vi "_CSMOFGV(lvlibp).vi"(6 "Operation":T7=enum."Get By Name", 7 "Allowed Messages (Empty For All)":string[](array[string]), 8 "Error In":errorcluster caption="error in (no error)", 9 "Mode":T1, 10 "Reference":string, 11 "Name (\"\" to Use UUID) In":string) -> (0 "error out":errorcluster, 1 "Boolean":bool, 3 "Array":T2[](array[typedef]))   [LabVIEW 2017, in "Communicable State Machine.lvlib"]
uses:
  Communicable State Machine.lvlib
  _CSMOFGVOPER.ctl
  _CSMObj.ctl
  _CSMObj-Info.ctl
  Typedef/_CSM_MODE.ctl
  _CSMObj-Refs.ctl
  _CSMObj-Data.ctl
  Typedef/_CSM_MSG_TYPE.ctl
  Priority Queue/Priority Queue.ctl
  Typedef/_Cross CSM State Data.ctl
  Typedef/_Cross CSM State Response.ctl
  Typedef/_CSM_Response Source Message.ctl
  Priority Queue/def-Data(LowPRI-Q).ctl
  _CSMObj-ModeData.ctl
  Typedef/_CSM Status Change Event Data.ctl
  Typedef/_CSM_List Module Scope.ctl
  _CSMOFGV.vi
  _Shared/CSM Shared.lvlib
panel:
  out "data":path
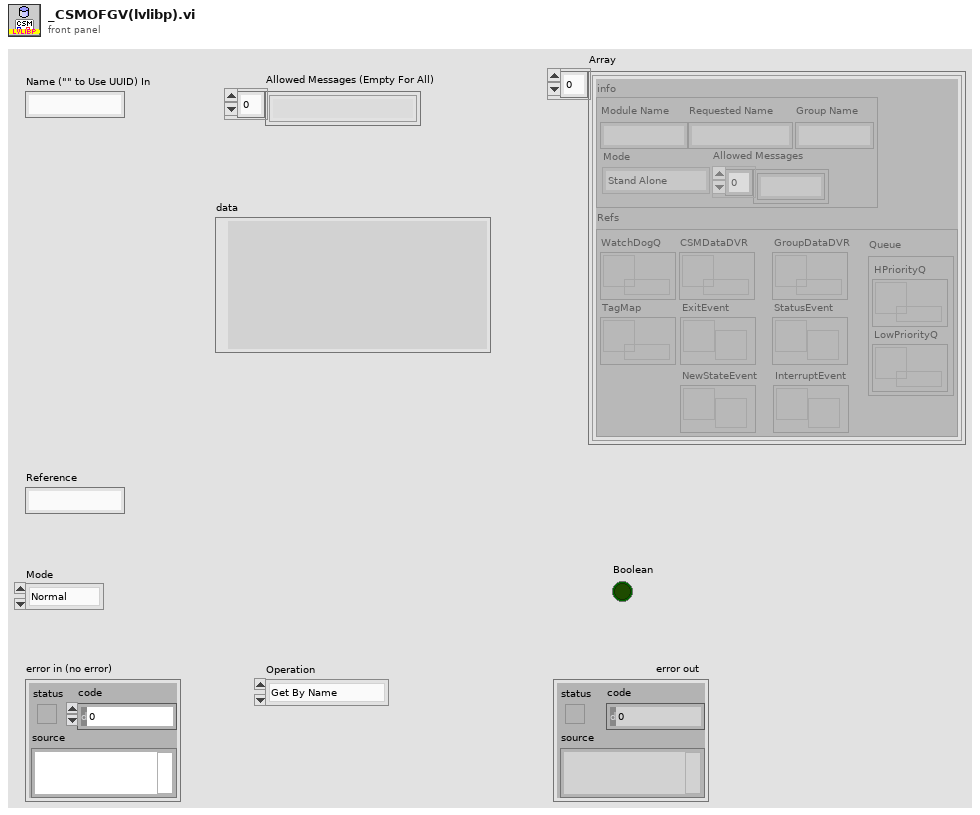
[diagram p1: front panel]
types:
  T1 = typedef "Communicable State Machine.lvlib/_CSM_List Module Scope.ctl" = enum16{"Normal", "System Only", "All"}
  T2 = typedef "Communicable State Machine.lvlib/_CSMObj.ctl" = cluster{"info":T3, "Refs":T5}
  T3 = typedef "Communicable State Machine.lvlib/_CSMObj-Info.ctl" = cluster{"Module Name":string, "Requested Name":string, "Group Name":string, "Mode":T4, "Allowed Messages":string[]}
  T4 = typedef "Communicable State Machine.lvlib/_CSM_MODE.ctl" = enum16{"Not Exist", "Stand Alone", "CSM", "Worker", "Worker Agent", "Chain Node", "Chain"}
  T5 = typedef "Communicable State Machine.lvlib/_CSMObj-Refs.ctl" = cluster{"WatchDogQ":refnum<queue>, "CSMDataDVR":refnum<data-value>, "Queue":T6, "GroupDataDVR":refnum<data-value>, "TagMap":refnum<data-value>, "ExitEvent":refnum<user-event>, "NewStateEvent":refnum<user-event>, "StatusEvent":refnum<user-event>, "InterruptEvent":refnum<user-event>}
  T6 = typedef "Communicable State Machine.lvlib/Priority Queue.ctl" = cluster{"HPriorityQ":refnum<queue>, "LowPriorityQ":refnum<queue>}
  T7 = typedef "Communicable State Machine.lvlib/_CSMOFGVOPER.ctl" = enum16{"Create If not Exist", "Get By Name", "List", "Check If Name Exists", "Release", "Module Status", "Create Status Event Handler", "Destroy Status Event Handler", "Clear Invalid Objs"}
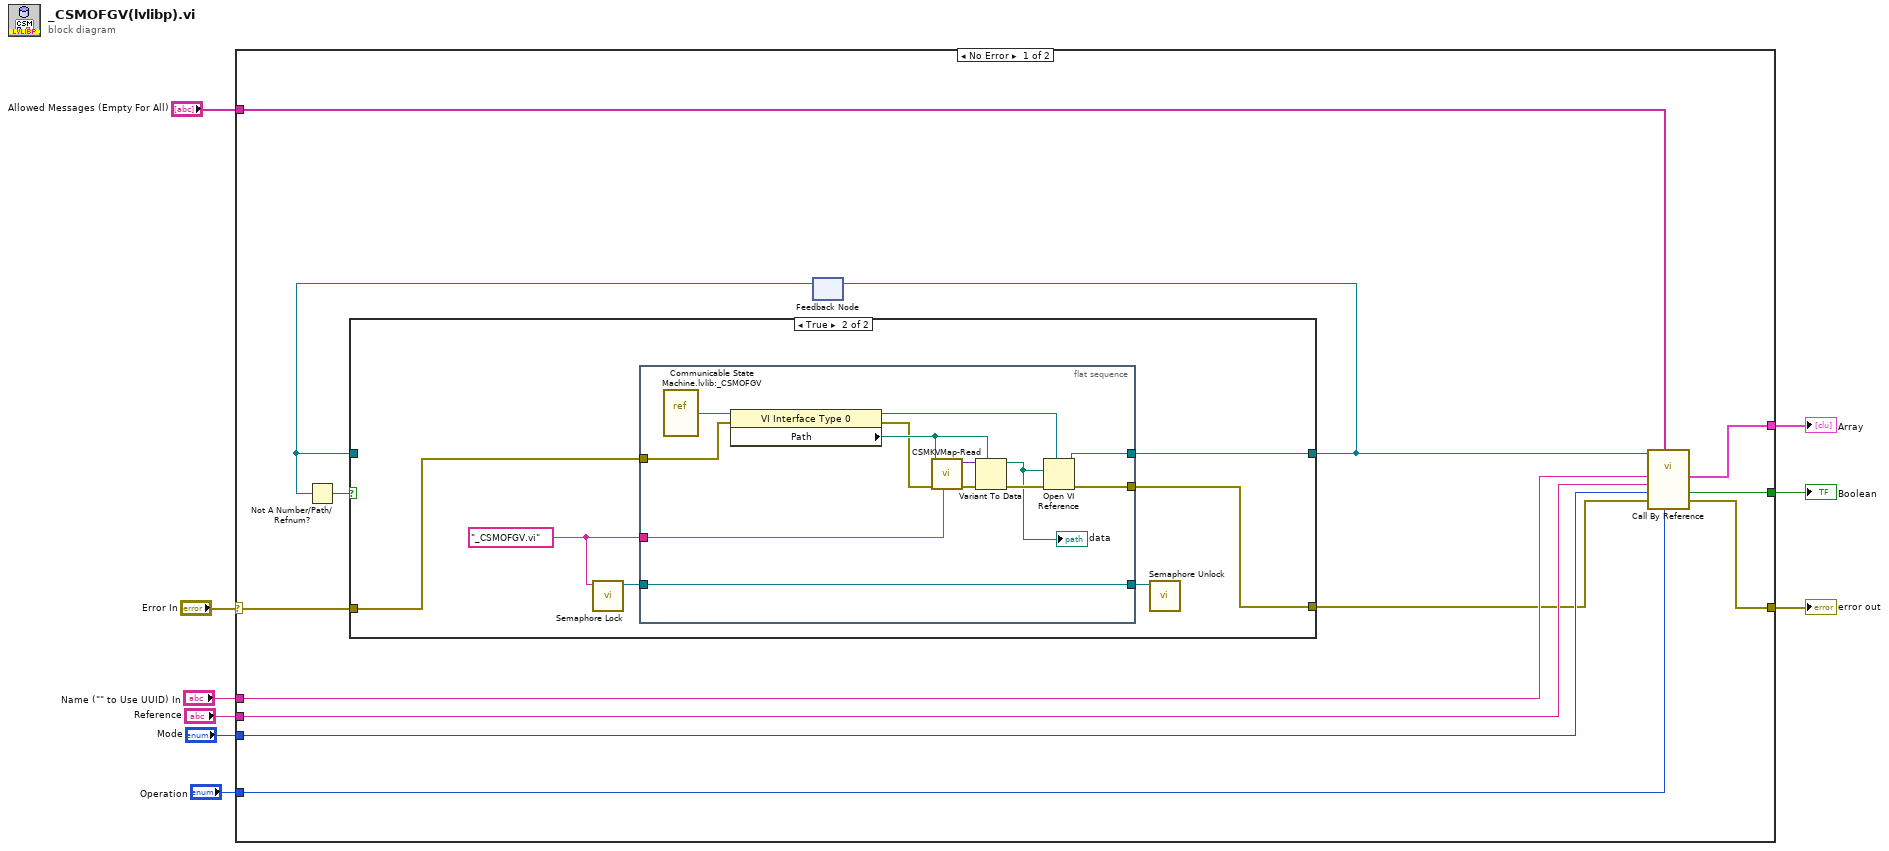
[diagram p0: block diagram]
diagram:
  n1 = case shown="No Error" "Error In" {
    selector: "Error In" -> [w11 w44]
    tunnel: [w19 _] -> w9
    tunnel: [w18 _] -> w8
    tunnel: [w17 w44] -> w7
    tunnel: "Allowed Messages (Empty For All)" -> [w16 _]
    tunnel: "Operation" -> [w15 _]
    tunnel: "Reference" -> [w14 _]
    tunnel: "Name (\"\" to Use UUID) In" -> [w13 _]
    tunnel: "Mode" -> [w12 _]
    frame No Error {
      n2 = feedback #1() -> (w21:refnum<vi>)  [unwired: 1 in]
      n3 = Not A Number/Path/Refnum?(number/path/refnum=w21) -> (NaN/Path/Refnum?=w22:bool)
      n4 = case shown="True" w22 {
        tunnel: [w24 w30] -> w20
        tunnel: w21 -> [w24 _]
        tunnel: w11 -> [w23 w28]
        tunnel: [w23 w27] -> w10
        frame False {
        }
        frame True {
          w29 = "_CSMOFGV.vi" ("name")
          n5 = call "Semaphore Lock.vi"("name"=w29) -> ("semaphore"=w25:refnum<queue>)  [unwired: 10 in]
          n6 = flat-sequence {
            tunnel: [w39] -> w30
            tunnel: w29 -> [w34]
            tunnel: w28 -> [w33]
            tunnel: [w32] -> w27
            tunnel: [w31] -> w26
            tunnel: w25 -> [w31]
            frame #0 {
              n7 = vi-ref "Communicable State Machine.lvlib:_CSMOFGV.vi"() -> (w38:refnum<vi>)
              n8 = property class="VI Interface Type 0"(reference=w38, error in=w33) -> (reference out=w37:refnum<vi>, error out=w36:errorcluster, "Path"=w40:path)
              n9 = call "CSMKVMap-Read.vi"("name"=w34, "Error in"=w36, "default value (empty variant)"=w40) -> ("Error out"=w43:errorcluster, "value"=w42:variant)  [unwired: 5 in]
              n10 = Variant To Data(error in=w43, type=w40, Variant=w42) -> (data=w35:path, error out=w41:errorcluster)
              "data" <- w35
              n11 = Open VI Reference(type specifier VI Refnum (for type only)=w37, vi path=w35, error in (no error)=w41) -> (vi reference=w39:refnum<vi>, error out=w32:errorcluster)  [unwired: 3 in]
            }
          }
          n12 = call "Semaphore Unlock.vi"("semaphore"=w26) -> ()  [unwired: 11 in]
        }
      }
      n13 = feedback-in #1(w20) -> ()
      n14 = call-by-ref "?"(reference=w20, "Operation"=w15, "Allowed Messages (Empty For All)"=w16, "Error In"=w10, "Mode"=w12, "Reference"=w14, "Name (\"\" to Use UUID) In"=w13) -> ("error out"=w17:errorcluster, "Boolean"=w18:bool, "Array"=w19:T2[])  [unwired: 4 in, 2 out]
    }
    frame Error {
    }
  }
  "error out" <- w7
  "Array" <- w9
  "Boolean" <- w8
